vi "LMS_GetDeviceList.vi"(8 "error in (no error)":errorcluster) -> (0 "error out":errorcluster, 1 "lms_info_str_t":string, 3 "Number of Devices":i32)   [LabVIEW 2013, in "LMS_LV_Drv.lvlib"]
uses:
  LMS_LV_Drv.lvlib
  LimeSuite.dll
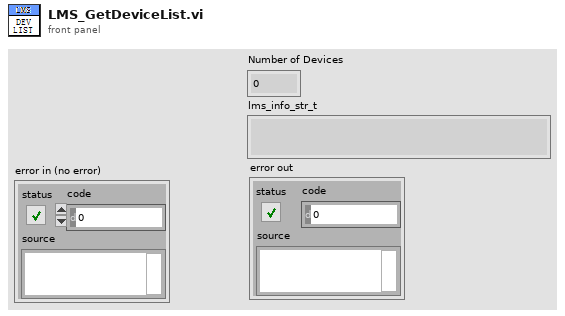
[diagram p1: front panel]
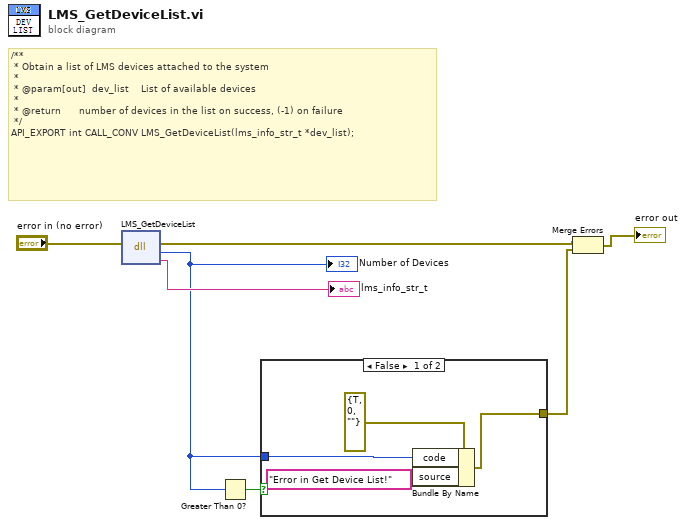
[diagram p0: block diagram]
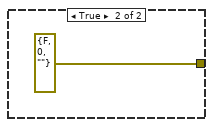
[diagram p2: hidden frame]
diagram:
  # "/**\n * Obtain a list of LMS devices attached to the system\n *\n * @param[out]  dev_list    List of available devices\n *\n * @return      number of devices in the list on success, (-1) on failure\n */\nAPI_EXPORT int CALL_CONV LMS_GetDeviceList(lms_info_str_t *dev_list);"
  n1 = dll-call lib="PTH1mabs CUsersOTADesktop书籍出版程序8.第八章LimeSDR_LabVIEW_Driver-master\nLimeSuite.dll" fn="LMS_GetDeviceList"(error in="error in (no error)") -> (error out=w4:errorcluster, "return type"=w1:i32, "lms_info_str_t"=→"lms_info_str_t":string)  [unwired: 3 in, 1 out]
  "Number of Devices" <- w1
  n2 = Greater Than 0?(x=w1) -> (x > 0?=w5:bool)
  n3 = case shown="False" w5 {
    tunnel: [w10 errorcluster {"status"=FALSE, "code"=0, "source"=""} ("error in")] -> w3
    tunnel: w1 -> [w9 _]
    frame False {
      n4 = Bundle By Name(cluster=errorcluster {"status"=TRUE, "code"=0, "source"=""} ("error in"), "code"=w9, "source"="Error in Get Device List!") -> (w10:errorcluster)
    }
    frame True {
    }
  }
  n5 = Merge Errors(w4, w3) -> (→"error out":errorcluster)
